vi "Harvester_1_26.vi"(0 "LimitSwitchIn":bool, 4 "LimitSwitchOut":bool, 8 "BallInHarv":bool, 9 "HarvInPos":dbl, 10 "HarvOutPos":dbl, 11 "HarvPot":dbl) -> (2 "HarvRoller":dbl, 3 "HarvPower":dbl)   [LabVIEW 2013]
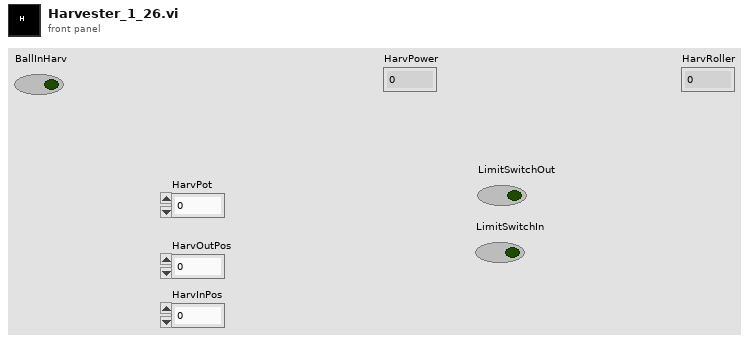
[diagram p1: front panel]
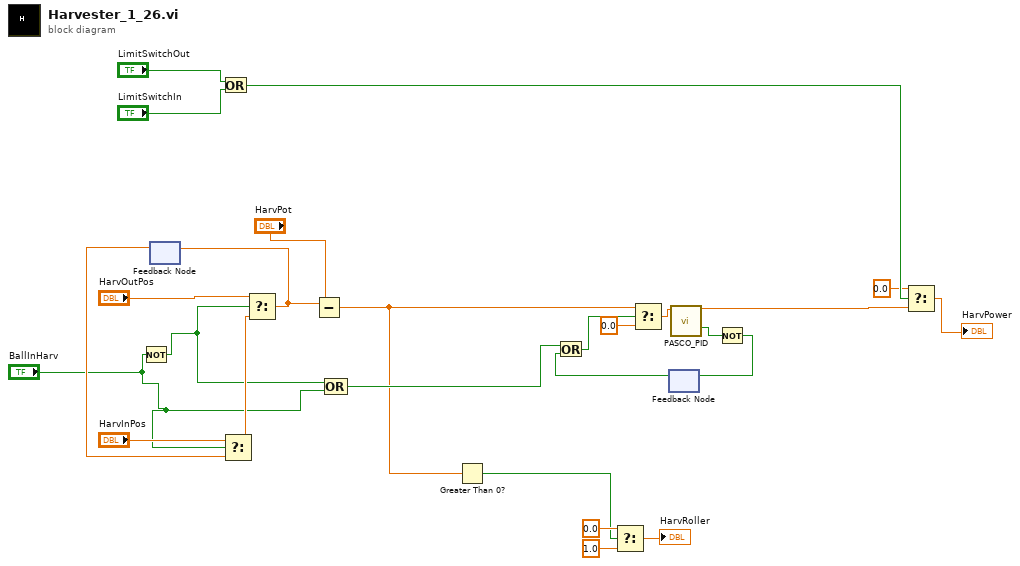
[diagram p0: block diagram]
diagram:
  n1 = Not(x="BallInHarv") -> (.not. x?=w2:bool)
  n2 = feedback #1() -> (w25:dbl)  [unwired: 1 in]
  n3 = Or(x="LimitSwitchOut", y="LimitSwitchIn") -> (x .or. y?=w19:bool)
  n4 = Select(t="HarvInPos", s="BallInHarv", f=w25) -> (s? t:f=w26:dbl)
  n5 = Select(t="HarvOutPos", s=w2, f=w26) -> (s? t:f=w24:dbl)
  n6 = feedback-in #1(w24) -> ()
  n7 = Subtract(x=w24, y="HarvPot") -> (x-y=w5:dbl)
  n8 = Compound Arithmetic op=OR(w2, "BallInHarv") -> (w11:bool)
  n9 = Greater Than 0?(x=w5) -> (x > 0?=w4:bool)
  n10 = Select(t=0.0, s=w4, f=1.0) -> (s? t:f=→"HarvRoller":dbl)
  n11 = feedback #2() -> (w9:bool)  [unwired: 1 in]
  n12 = Or(x=w11, y=w9) -> (x .or. y?=w10:bool)
  n13 = Select(t=w5, s=w10, f=0.0) -> (s? t:f=w21:dbl)
  n14 = call "PASCO_PID.vi"("Delta"=w21) -> ("Output"=w18:dbl, "IsThere"=w3:bool)  [unwired: 13 in]
  n15 = Not(x=w3) -> (.not. x?=w20:bool)
  n16 = feedback-in #2(w20) -> ()
  n17 = Select(t=0.0, s=w19, f=w18) -> (s? t:f=→"HarvPower":dbl)
